vi "InstrumentBase_Init.vi"(0 "object in":refnum<class "InstrumentBase.lvclass">, 5 "error in (no error)":errorcluster) -> (14 "object out":refnum<class "InstrumentBase.lvclass">, 19 "error out":errorcluster)   [LabVIEW 2019, in "InstrumentBase.lvclass"]
uses:
  InstrumentBase.lvclass
  InstrumentBase.lvclass/InstrumentBase.ctl
panel:
  in  "MinAmplitude":dbl
  in  "MaxAmplitude":dbl=10.0
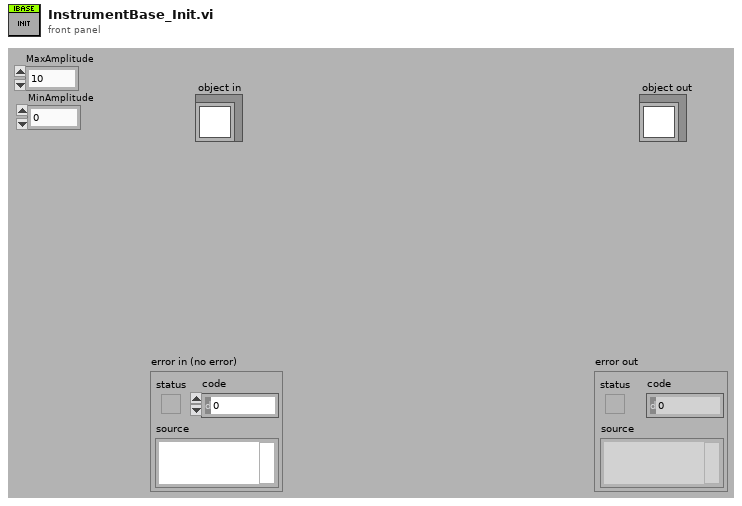
[diagram p1: front panel]
types:
  T1 = cluster{"Message":string, "Message Data":variant}
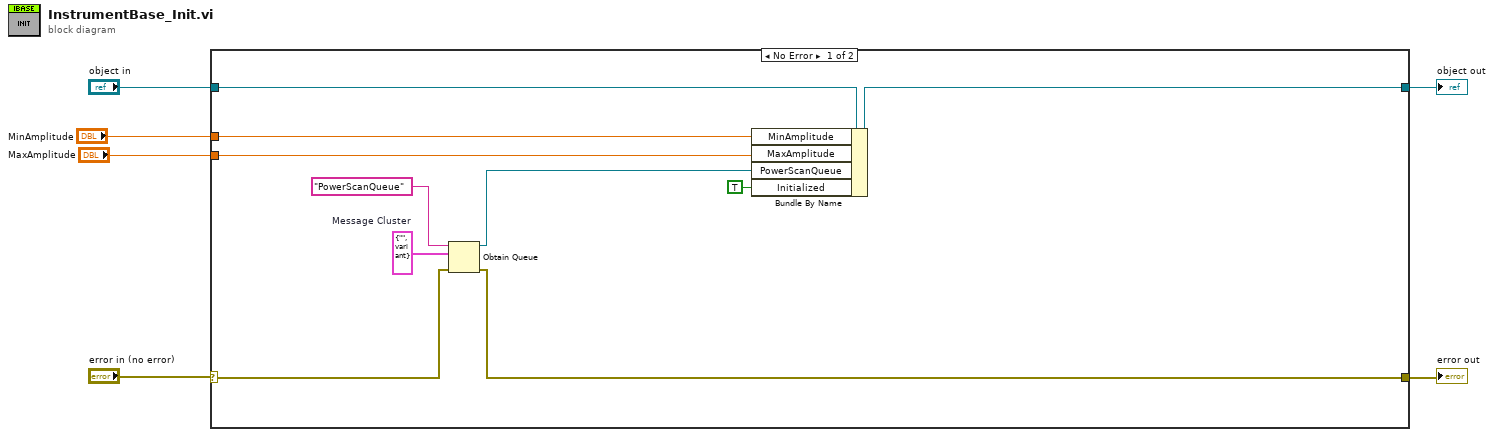
[diagram p0: block diagram]
diagram:
  n1 = case shown="No Error" "error in (no error)" {
    selector: "error in (no error)" -> [w14 w17]
    tunnel: "object in" -> [w16 w18]
    tunnel: [w12 w18] -> w5
    tunnel: [w13 w17] -> w3
    tunnel: "MaxAmplitude" -> [w9 _]
    tunnel: "MinAmplitude" -> [w8 _]
    frame No Error {
      w15 = T1 {"Message"="", "Message Data"=variant}  # Message Cluster
      n2 = Obtain Queue(name (unnamed)="PowerScanQueue", element data type=w15, error in (no error)=w14) -> (queue out=w11:refnum<queue>, error out=w13:errorcluster)  [unwired: 2 in, 1 out]
      n3 = Bundle By Name(cluster=w16, "MinAmplitude"=w8, "MaxAmplitude"=w9, "PowerScanQueue"=w11, "Initialized"=TRUE) -> (w12:refnum<class "InstrumentBase.lvclass">)
    }
    frame Error {
    }
  }
  "object out" <- w5
  "error out" <- w3
